vi "DmgrGetDvc.vi"(8 "Error In":errorcluster, 11 "Device Number":i32) -> (0 "Error Out":errorcluster)   [LabVIEW 2011, in "LVH-Adept.lvlib" / "DMGR.lvlib"]
doc: "Get Device Handle"
uses:
  DMGR.lvlib
  Type Defs/Error Type.ctl
  LVH-Adept.lvlib
  Resources/dmgr.dll
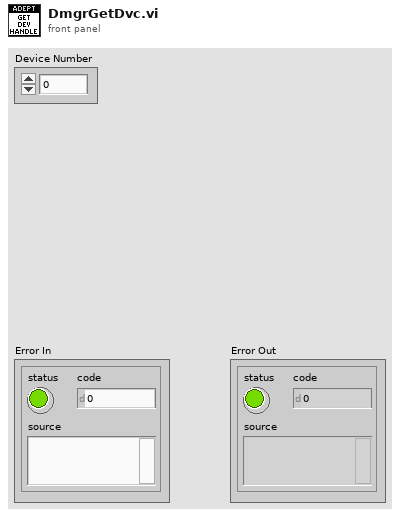
[diagram p1: front panel]
types:
  T1 = typedef "LVH-Adept.lvlib/Error Type.ctl" = enum16{"Unknown Error", "Device Enumeration", "Device Handle", "Device Info"}
  T2 = cluster{"[0]":u8, "[1]":u8, "[2]":u8, "[3]":u8, "[4]":u8, "[5]":u8, "[6]":u8, "[7]":u8, "[8]":u8, "[9]":u8, "[10]":u8, "[11]":u8, "[12]":u8, "[13]":u8, "[14]":u8, "[15]":u8}
  T3 = cluster{u8[], u8[], cluster{"[0]":u8, "[1]":u8, "[2]":u8, "[3]":u8, "[4]":u8, "[5]":u8, "[6]":u8, "[7]":u8, "[8]":u8, "[9]":u8, "[10]":u8, "[11]":u8, "[12]":u8, "[13]":u8, "[14]":u8, "[15]":u8}}
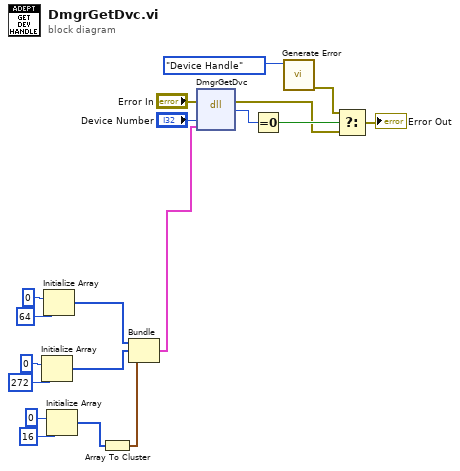
[diagram p0: block diagram]
diagram:
  n1 = Initialize Array(u8 0 ("element"), 272 ("dimension size")) -> (w4:u8[])
  n2 = Initialize Array(u8 0 ("element"), 64 ("dimension size")) -> (w5:u8[])
  n3 = Initialize Array(u8 0 ("element"), 16 ("dimension size")) -> (w3:u8[])
  n4 = Array To Cluster(array=w3) -> (cluster=w2:T2)
  n5 = Bundle(w5, w4, w2) -> (w1:T3)  [unwired: 1 in]
  n6 = dll-call lib="C:/github/labviewhacker/LVH-Adept/LabVIEW/vi.lib/LabVIEW Hacker/Adept/Private/Resources/dmgr.dll" fn="DmgrGetDvc"(error in="Error In", "Device Number"="Device Number", "Device Handle *"=w1) -> (error out=w13:errorcluster, "Error?"=w18:i8)  [unwired: 4 in, 1 out]
  n7 = Equal To 0?(x=w18) -> (x = 0?=w17:bool)
  n8 = call "Generate Error.vi"("Error Type"=Error_Type."Device Handle") -> ("Error Out"=w14:errorcluster)  [unwired: 10 in]
  n9 = Select(t=w14, s=w17, f=w13) -> (s? t:f=→"Error Out":errorcluster)
